vi "LOGregister.vi"(7 "Maximum Messages":i32, 8 "Error In":errorcluster, 10 "Listener ID":string, 11 "Listeners In":refnum<queue>[](array[refnum])) -> (0 "Error Out":errorcluster, 3 "Listeners Out":refnum<queue>[](array[refnum]))   [LabVIEW 2025]
uses:
  LOGstatement.ctl
  <vilib>/Field R&D Services/Logger/Type Definitions/Tag.ctl
  <vilib>/Field R&D Services/Logger/Field_RnD_Services_Logger_Toolkit.lvlib
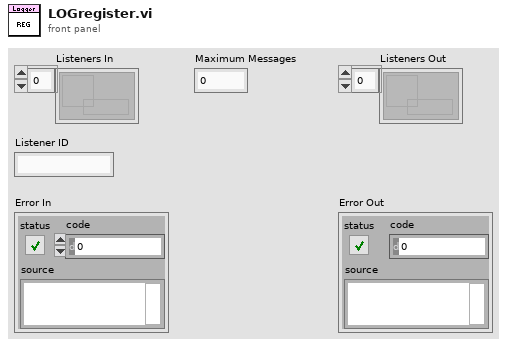
[diagram p1: front panel]
types:
  T1 = typedef "Field_RnD_Services_Logger_Toolkit.lvlib/LOGstatement.ctl" = cluster{"Time Stamp":timestamp, "Tag":T2, "Source":string, "Message":string}
  T2 = typedef "Field_RnD_Services_Logger_Toolkit.lvlib/Tag.ctl" = enum16{"Fatal", "Error", "Warn", "Info", "Debug", "Trace"}
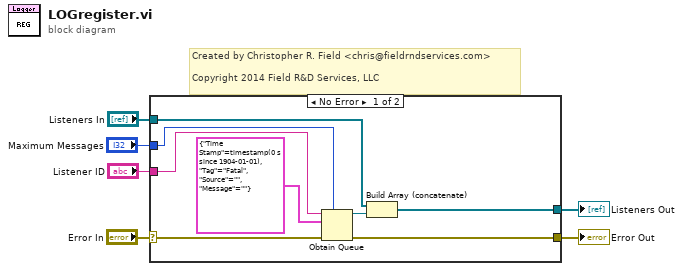
[diagram p0: block diagram]
diagram:
  # "Created by Christopher R. Field <chris@fieldrndservices.com>\n\nCopyright 2014 Field R&D Services, LLC"
  n1 = case shown="No Error" "Error In" {
    selector: "Error In" -> [w11 w16]
    tunnel: "Listener ID" -> [w9 _]
    tunnel: "Listeners In" -> [w14 w15]
    tunnel: [w13 w15] -> w4
    tunnel: [w10 w16] -> w3
    tunnel: "Maximum Messages" -> [w7 _]
    frame No Error {
      n2 = Obtain Queue(max queue size (-1, unlimited)=w7, name (unnamed)=w9, element data type=T1 {"Time Stamp"=timestamp(0 s since 1904-01-01), "Tag"=enum."Fatal", "Source"="", "Message"=""} ("Message"), error in (no error)=w11) -> (queue out=w8:refnum<queue>, error out=w10:errorcluster)  [unwired: 1 in, 1 out]
      n3 = Build Array (concatenate)(w14, w8) -> (w13:refnum<queue>[])
    }
    frame Error {
    }
  }
  "Listeners Out" <- w4
  "Error Out" <- w3
